vi "Msg.Q.Enqueue.vi"(6 "Enqueue Mode":T1, 8 "Error (in)":errorcluster, 9 "Data":variant, 10 "Message":string, 11 "Msg.Q.Ref":T2) -> (0 "Error (out)":errorcluster, 3 "Msg.Q.Ref (out)":T2)   [LabVIEW 2023]
doc: "This VI is used to enqueu an element of message and data in a queue"
uses:
  Msg.Q.Ref.ctl
  Msg.Data.ctl
  Msg.Q.EnqueueMode.ctl
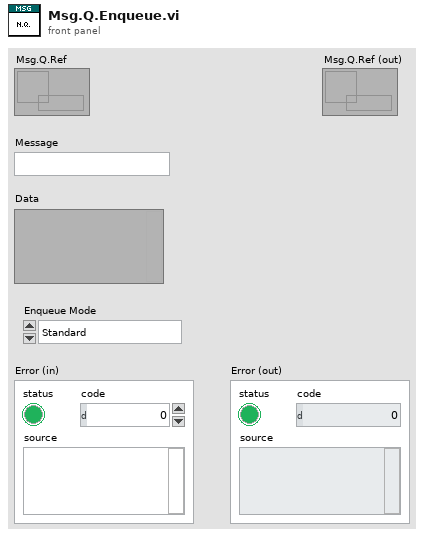
[diagram p1: front panel]
types:
  T1 = typedef "Msg.Q.EnqueueMode.ctl" = enum16{"Standard", "Lossy"}
  T2 = typedef "Msg.Q.Ref.ctl" = refnum<queue>
  T3 = typedef "Msg.Data.ctl" = cluster{"Message":string, "Data":variant}
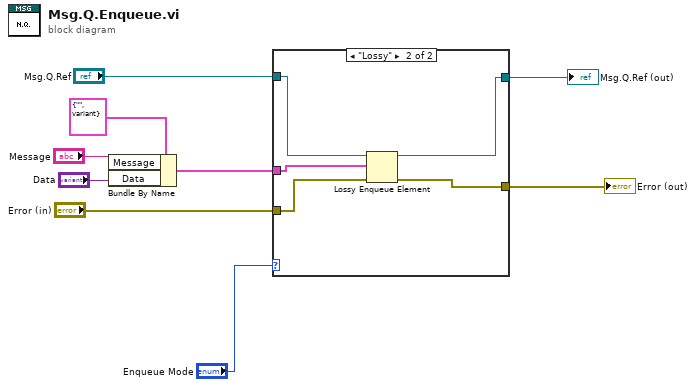
[diagram p0: block diagram]
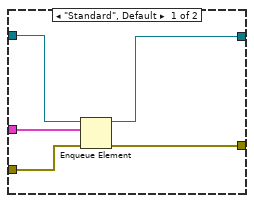
[diagram p2: hidden frame]
diagram:
  n1 = Bundle By Name(cluster=T3 {"Message"="", "Data"=variant} ("Msg.Q.Data"), "Message"="Message", "Data"="Data") -> (w2:T3)
  n2 = case shown="\"Lossy\"" "Enqueue Mode" {
    tunnel: "Msg.Q.Ref" -> [w14 w19]
    tunnel: "Error (in)" -> [w13 w17]
    tunnel: [w12 w15] -> w7
    tunnel: [w11 w16] -> w6
    tunnel: w2 -> [w10 w18]
    frame "Standard", Default {
      n3 = Enqueue Element(queue=w14, element=w10, error in (no error)=w13) -> (queue out=w12:T2, error out=w11:errorcluster)  [unwired: 1 in, 1 out]
    }
    frame "Lossy" {
      n4 = Lossy Enqueue Element(queue=w19, element=w18, error in (no error)=w17) -> (queue out=w15:T2, error out=w16:errorcluster)  [unwired: 2 out]
    }
  }
  "Msg.Q.Ref (out)" <- w7
  "Error (out)" <- w6
